vi "Read failed to connect.vi"(8 "error in":errorcluster, 11 "MQTT client in":refnum<class "MQTT client.lvclass">) -> (0 "error out":errorcluster, 3 "MQTT client out":refnum<class "MQTT client.lvclass">)   [LabVIEW 2014, in "MQTT client.lvclass"]
uses:
  MQTT client.lvclass
  status event.ctl
panel:
  out "failed to connect":refnum<event-registration>
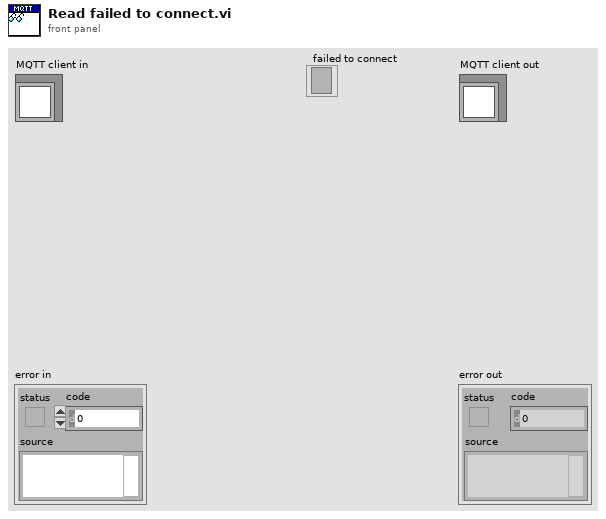
[diagram p1: front panel]
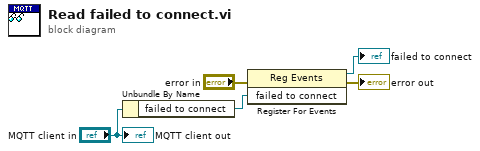
[diagram p0: block diagram]
diagram:
  n1 = Unbundle By Name("MQTT client in") -> ("failed to connect"=w2:refnum<user-event>)
  n2 = register-events(error in="error in", w2) -> (reference out=→"failed to connect":refnum<event-registration>, error out=→"error out":errorcluster)  [unwired: 1 in]
  "MQTT client out" <- "MQTT client in"
